vi "Team Index.vi"(11 "Team":refnum<class "Team.lvclass">) -> (2 "Team Index":i32)   [LabVIEW 2020, in "SquareBattle.lvlib" / "Team.lvclass"]
uses:
  Team.lvclass
  Team.lvclass/Team.ctl
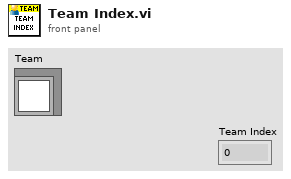
[diagram p1: front panel]
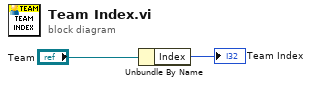
[diagram p0: block diagram]
diagram:
  n1 = Unbundle By Name("Team") -> ("Index"=→"Team Index":i32)
